vi "run script line.vi"(8 "error in (no error)":errorcluster caption="에러 입력(에러 없음)", 11 "Script Line_i2c r 입력":refnum<class "Script Line_i2c r.lvclass">) -> (0 "error out":errorcluster caption="에러 출력", 2 "log":string, 3 "Script Line_i2c r 출력":refnum<class "Script Line_i2c r.lvclass">)   [LabVIEW 2020, in "Script Line_i2c r.lvclass"]
uses:
  Script Line_i2c r.lvclass
  Script Line_i2c/Script Line_i2c.lvclass/Script Line_i2c.ctl
  Script Line_i2c/Accessors/Read reg.vi
  Script Line_i2c/Accessors/Read size.vi
  Script Line_i2c/Accessors/Read slv.vi
  Script Line_i2c/Accessors/Read reg addr byte.vi
  Script Line_i2c/Accessors/Write data.vi
  BD Protocol Class/I2C/I2C.lvclass
  Script Line_i2c/Script Line_i2c.lvclass
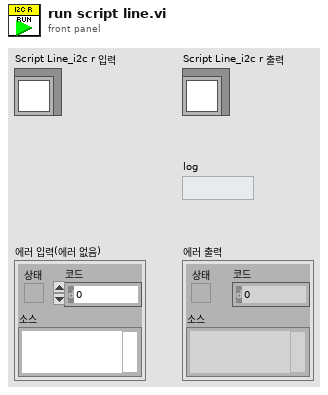
[diagram p1: front panel]
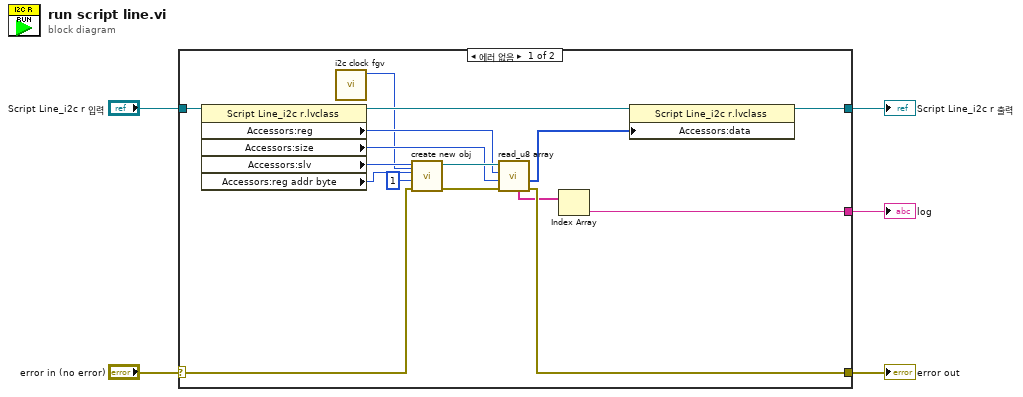
[diagram p0: block diagram]
diagram:
  n1 = case shown="에러 없음" "error in (no error)" {
    selector: "error in (no error)" -> [w18 w23]
    tunnel: [w17 w23] -> w2
    tunnel: [w15 w22] -> w4
    tunnel: "Script Line_i2c r 입력" -> [w16 w22]
    tunnel: [w8 _] -> w1
    frame No Error {
      n2 = property class="Script Line_i2c r.lvclass"(reference=w16) -> (reference out=w14:refnum<class "Script Line_i2c r.lvclass">, "Accessors:reg"=w13:u32, "Accessors:size"=w9:u32, "Accessors:slv"=w12:u8, "Accessors:reg addr byte"=w10:u8)  [unwired: 1 in, 1 out]
      n3 = call "i2c clock fgv.vi"() -> ("i2c clock out"=w7:u8)  [unwired: 10 in, 1 out]
      n4 = call "create new obj.vi"("clock rate"=w7, "error in (no error)"=w18, "data byte"=u8 1 ("address byte"), "address byte"=w10, "slave address"=w12) -> ("error out"=w19:errorcluster, "new I2C obj"=w20:refnum<class "I2C.lvclass">)  [unwired: 5 in]
      n5 = call-dynamic "read_u8 array.vi"("error in (no error)"=w19, "size to read"=w9, "start address"=w13, "I2C 입력"=w20) -> ("error out"=w17:errorcluster, "data out"=w11:u8[], "log_single line"=w6:string[])  [unwired: 3 in, 2 out]
      n6 = Index Array(array=w6) -> (element=w8:string)  [unwired: 1 in]
      n7 = property class="Script Line_i2c r.lvclass"(reference=w14, "Accessors:data"=w11) -> (reference out=w15:refnum<class "Script Line_i2c r.lvclass">)  [unwired: 1 in, 1 out]
    }
    frame Error {
    }
  }
  "error out" <- w2
  "Script Line_i2c r 출력" <- w4
  "log" <- w1
